vi "main.vi"() -> ()   [LabVIEW 2019]
doc: "This example performs writes and reads on a serial port, as directed by the user. You can press the Write and Read buttons, and change the Read Count, while the example is running.\n\nThe parameters set for the serial port must match the parameters of the connected instrument or device. In this example, the Read Count parameter specifies the number of bytes that the serial port reads. If there were more bytes at the port than the specified number, those bytes would not be read. If there were less bytes at the port than the specified number, you would receive a timeout error.\n\nThis example expands upon the flow control options for XON and XOFF, allowing the user to choose those control characters. Also, the user can enable or disable a termination character. Some devices require a termination character in order to identify the end of command strings. Some devices send a termination character to signify the end of data to be read. This example shows how you can end the Read operation once a termination character is detected in the buffer and/or append a termination character at the end of the Write data."
uses:
  type_cmd.ctl
  type_rxmsg.ctl
panel:
  out "Array":T1[](array[typedef])
  out "stopped":bool=TRUE
  in  "mac2connect":u8[](array[numeric])=[135, 0, 48, 218, 24, 0] format="0x%x"
  in  "cmd":bool
  out "raw cmd":string
  in  "payload":u8[](array[numeric])=[65, 66, 67, 68] format="0x%x"
  in  "command":T2=enum."connect"
  in  "Stop":bool
  in  "VISA resource name":refnum<visa-resource-name>="COM1"
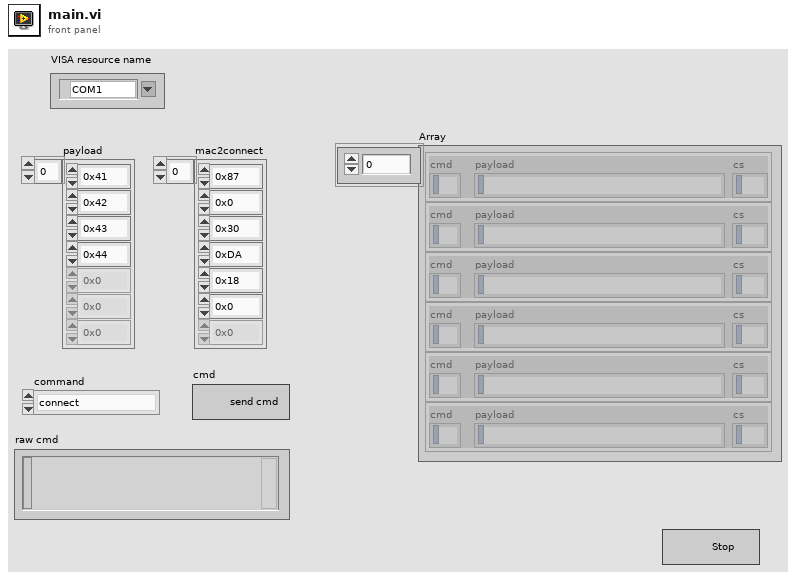
[diagram p1: front panel]
types:
  T1 = typedef "type_rxmsg.ctl" = cluster{"cmd":string, "payload":string, "cs":string}
  T2 = typedef "type_cmd.ctl" = enum16{"setting_factoryreset", "setting_justworks", "scan_getdevices", "scan_stop", "scan_start", "send", "disconnect", "connect"}
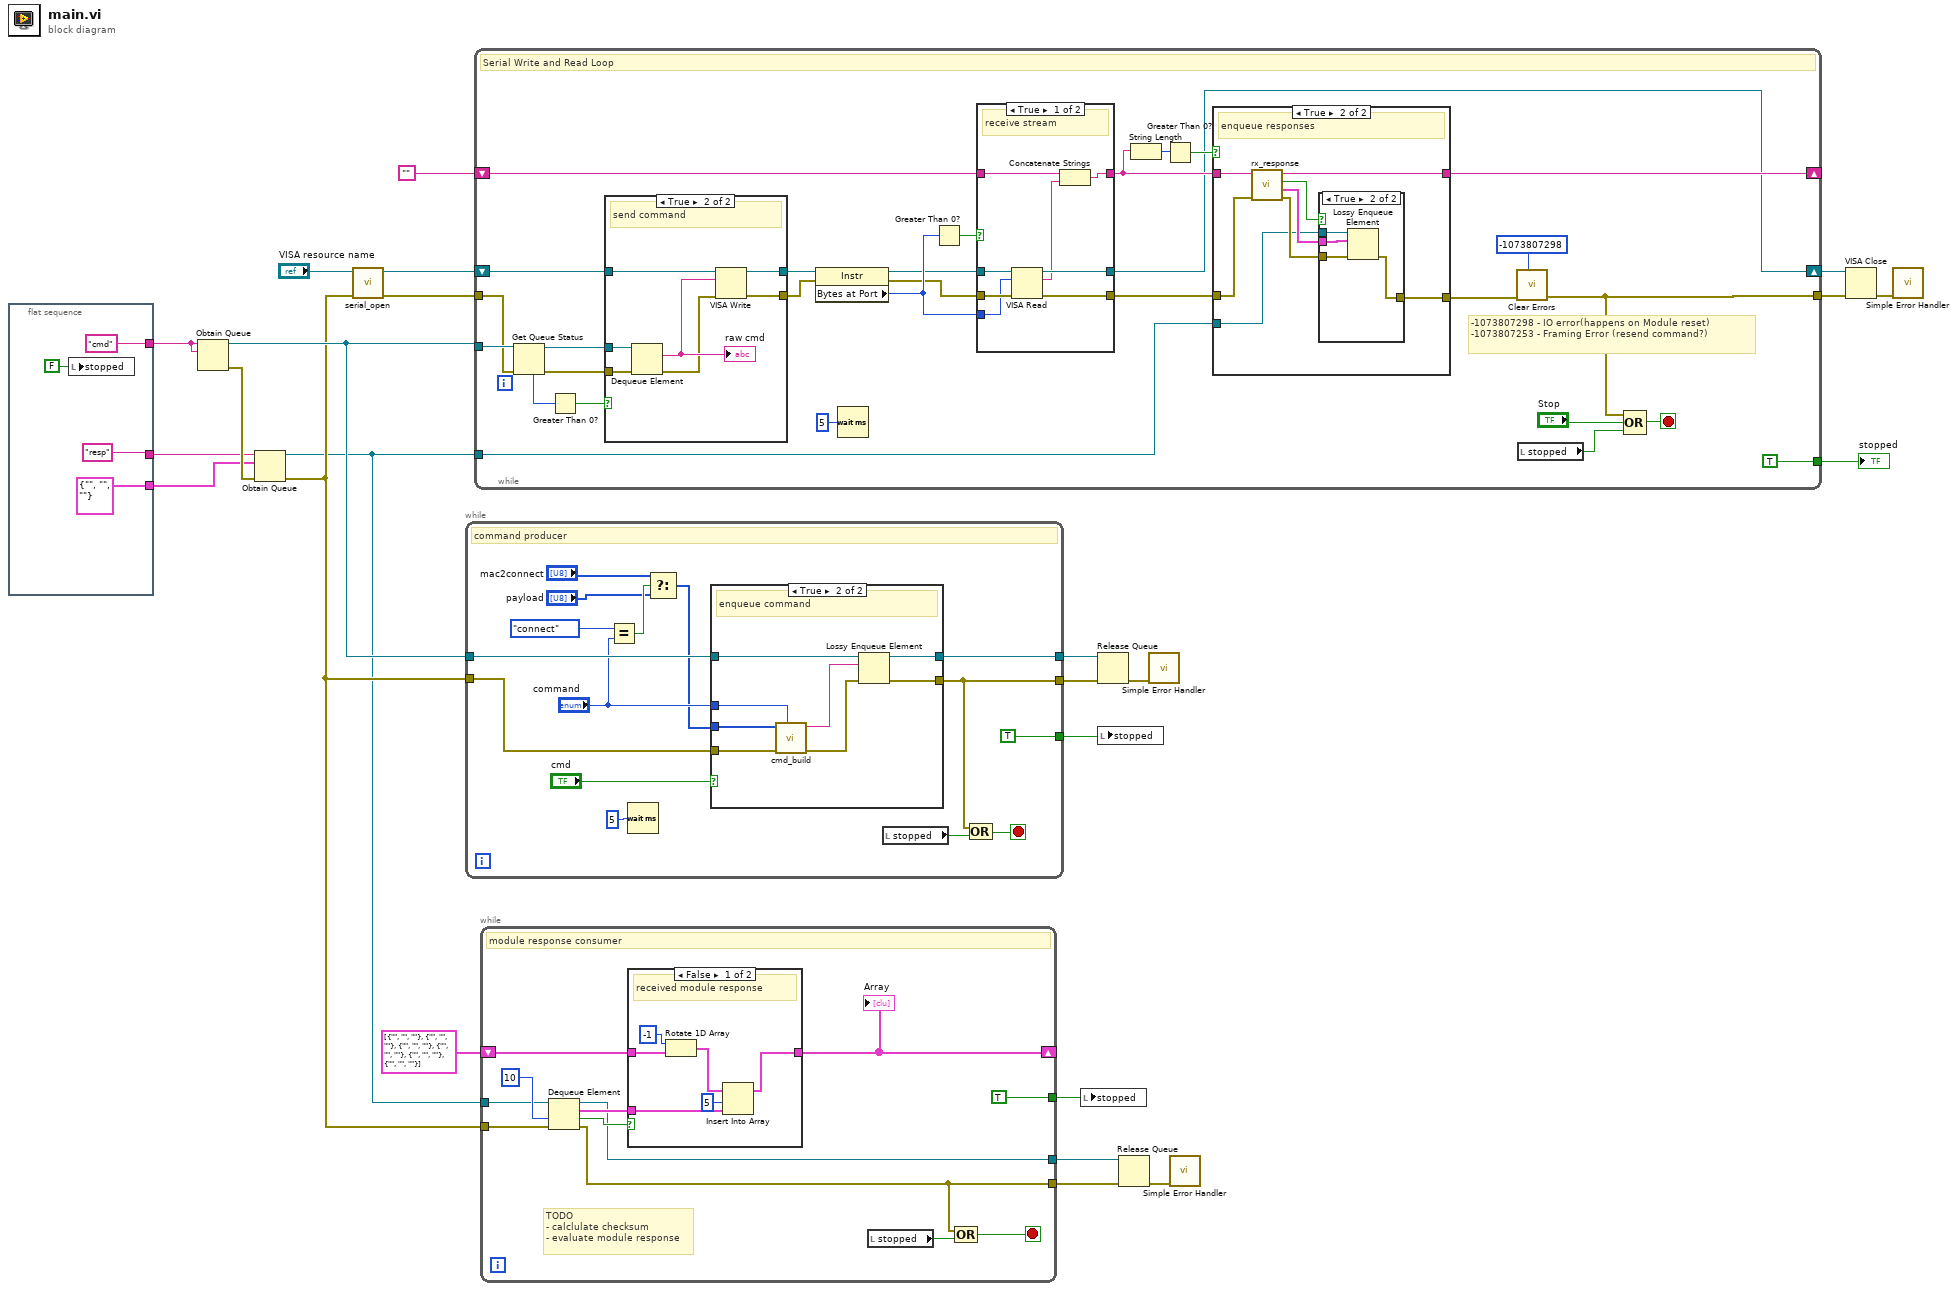
[diagram p0: block diagram]
diagram:
  n1 = flat-sequence {
    tunnel: ["cmd" ("name (unnamed)")] -> w11
    tunnel: ["resp" ("name (unnamed)")] -> w9
    tunnel: [T1 {"cmd"="", "payload"="", "cs"=""} ("rx msg")] -> w8
    frame #0 {
      n2 = local write "stopped"(FALSE ("stopped")) -> ()
    }
  }
  n3 = Obtain Queue(name (unnamed)=w11, element data type=w11) -> (queue out=w15:refnum<queue>, error out=w10:errorcluster)  [unwired: 3 in, 1 out]
  n4 = Obtain Queue(name (unnamed)=w9, element data type=w8, error in (no error)=w10) -> (queue out=w6:refnum<queue>, error out=w7:errorcluster)  [unwired: 2 in, 1 out]
  n5 = call "serial_open.vi"("error in"=w7, "VISA Refnum in"="VISA resource name") -> ("error out"=w20:errorcluster, "VISA Refnum out"=w19:refnum<visa-resource-name>)  [unwired: 8 in]
  n6 = while {
    tunnel: w15 -> [w43]
    tunnel: [w42] -> w18
    tunnel: [w31] -> w17
    tunnel: w7 -> [w41]
    tunnel: [TRUE] -> w12
    stop <- w32 stop-if-true
    # "command producer"
    n7 = Equal?(x=type_cmd."connect" ("command"), y="command") -> (x = y?=w36:bool)
    n8 = Wait (ms)(milliseconds to wait=u32 5) -> ()  [unwired: 1 out]
    n9 = Select(t="mac2connect", s=w36, f="payload") -> (s? t:f=w33:u8[])
    n10 = case shown="True" "cmd" {
      tunnel: w43 -> [w45 w52]
      tunnel: [w45 w53] -> w42
      tunnel: "command" -> [_ w50]
      tunnel: [w44 w48] -> w31
      tunnel: w41 -> [w44 w47]
      tunnel: w33 -> [_ w46]
      frame False {
      }
      frame True {
        # "enqueue command"
        n11 = call "cmd_build.vi"("command"=w50, "error  in"=w47, "payload"=w46) -> ("out"=w49:errorcluster, "cmd"=w51:string)  [unwired: 7 in]
        n12 = Lossy Enqueue Element(queue=w52, element=w51, error in (no error)=w49) -> (queue out=w53:refnum<queue>, error out=w48:errorcluster)  [unwired: 2 out]
      }
    }
    n13 = local read "stopped"() -> (w30:bool)
    n14 = Compound Arithmetic op=OR(w31, w30) -> (w32:bool)
  }
  n15 = while {
    shift-right: [w54] -> w21
    shift-left: w19 -> [w82]
    tunnel: w20 -> [w73]
    tunnel: [w66] -> w22
    tunnel: w15 -> [w77]
    tunnel: [TRUE] -> w14
    shift-right: [w55] -> _
    shift-left: "" -> [w62]
    tunnel: w6 -> [w57]
    stop <- w63 stop-if-true
    # "-1073807298 - IO error(happens on Module reset)\n-1073807253 - Framing Error (resend command?)"
    # "Serial Write and Read Loop"
    n16 = Get Queue Status(queue=w77, error in (no error)=w73) -> (queue out=w74:refnum<queue>, error out=w72:errorcluster, # elements in queue=w76:i32)  [unwired: 1 in, 5 out]
    n17 = Greater Than 0?(x=w76) -> (x > 0?=w75:bool)
    n18 = case shown="True" w75 {
      tunnel: w82 -> [w99 w106]
      tunnel: [w99 w105] -> w69
      tunnel: [w98 w104] -> w71
      tunnel: w74 -> [_ w103]
      tunnel: w72 -> [w98 w101]
      frame False {
      }
      frame True {
        # "send command"
        n19 = Dequeue Element(queue=w103, error in (no error)=w101) -> (element=w102:string, error out=w100:errorcluster)  [unwired: 1 in, 2 out]
        "raw cmd" <- w102
        n20 = VISA Write(VISA resource name=w106, write buffer=w102, error in (no error)=w100) -> (VISA resource name out=w105:refnum<visa-resource-name>, error out=w104:errorcluster)  [unwired: 1 out]
      }
    }
    n21 = property class="Instr"(reference=w69, error in=w71) -> (reference out=w68:refnum<visa-resource-name>, error out=w70:errorcluster, "Bytes at Port"=w79:u32)
    n22 = Wait (ms)(milliseconds to wait=u32 5) -> ()  [unwired: 1 out]
    n23 = Greater Than 0?(x=w79) -> (x > 0?=w80:bool)
    n24 = case shown="True" w80 {
      tunnel: [w112 w117] -> w54
      tunnel: w68 -> [w114 w117]
      tunnel: w70 -> [w113 w115]
      tunnel: w79 -> [w111 _]
      tunnel: w62 -> [w110 w116]
      tunnel: [w108 w116] -> w60
      tunnel: [w107 w115] -> w61
      frame True {
        # "receive stream"
        n25 = VISA Read(VISA resource name=w114, byte count=w111, error in (no error)=w113) -> (VISA resource name out=w112:refnum<visa-resource-name>, read buffer=w109:string, error out=w107:errorcluster)  [unwired: 1 out]
        n26 = Concatenate Strings(w110, w109) -> (w108:string)
      }
      frame False {
      }
    }
    n27 = String Length(string=w60) -> (length=w59:i32)
    n28 = Greater Than 0?(x=w59) -> (x > 0?=w58:bool)
    n29 = case shown="True" w58 {
      tunnel: [w83 w90] -> w55
      tunnel: w61 -> [w84 w92]
      tunnel: w60 -> [w83 w91]
      tunnel: w57 -> [_ w86]
      tunnel: [w84 w85] -> w56
      frame False {
      }
      frame True {
        # "enqueue responses"
        n30 = call "rx_response.vi"("error in"=w92, "msg in"=w91) -> ("error out"=w87:errorcluster, "rx msg"=w88:T1, "msg complete"=w89:bool, "remain"=w90:string)  [unwired: 6 in]
        n31 = case shown="True" w89 {
          tunnel: w88 -> [_ w97]
          tunnel: w87 -> [w93 w96]
          tunnel: w86 -> [_ w95]
          tunnel: [w93 w94] -> w85
          frame False {
          }
          frame True {
            n32 = Lossy Enqueue Element(queue=w95, element=w97, error in (no error)=w96) -> (error out=w94:errorcluster)  [unwired: 3 out]
          }
        }
      }
    }
    n33 = call <vilib>:"Clear Errors.vi"("error in (no error)"=w56, "specific error code to clear (0: all)"=-1073807298) -> ("error out"=w66:errorcluster)  [unwired: 4 in, 1 out]
    n34 = local read "stopped"() -> (w64:bool)
    n35 = Compound Arithmetic op=OR(w66, "Stop", w64) -> (w63:bool)
  }
  "stopped" <- w14
  n36 = while {
    tunnel: w7 -> [w127]
    tunnel: w6 -> [w126]
    shift-right: [w123] -> _
    shift-left: T1[] [{"cmd"="", "payload"="", "cs"=""}, {"cmd"="", "payload"="", "cs"=""}, {"cmd"="", "payload"="", "cs"=""}, {"cmd"="", "payload"="", "cs"=""}, {"cmd"="", "payload"="", "cs"=""}, {"cmd"="", "payload"="", "cs"=""}] -> [w124]
    tunnel: [w121] -> w3
    tunnel: [w120] -> w2
    tunnel: [TRUE] -> w1
    stop <- w119 stop-if-true
    # "TODO \n- calclulate checksum\n- evaluate module response"
    # "module response consumer"
    n37 = Dequeue Element(queue=w126, timeout in ms (-1)=10, error in (no error)=w127) -> (queue out=w121:refnum<queue>, element=w122:T1, timed out?=w125:bool, error out=w120:errorcluster)
    n38 = case shown="False" w125 {
      tunnel: w124 -> [w135 w136]
      tunnel: [w131 w136] -> w123
      tunnel: w122 -> [w130 _]
      frame False {
        # "received module response"
        n39 = Rotate 1D Array(1:w135, 2:-1 ("n")) -> (0:w132:T1[])
        n40 = Insert Into Array(array=w132, index=5, new element=w130) -> (w131:T1[])
      }
      frame True {
      }
    }
    "Array" <- w123
    n41 = local read "stopped"() -> (w128:bool)
    n42 = Compound Arithmetic op=OR(w120, w128) -> (w119:bool)
  }
  n43 = local write "stopped"(w1) -> ()
  n44 = Release Queue(queue=w18, error in (no error)=w17) -> (error out=w16:errorcluster)  [unwired: 1 in, 2 out]
  n45 = local write "stopped"(w12) -> ()
  n46 = Release Queue(queue=w3, error in (no error)=w2) -> (error out=w4:errorcluster)  [unwired: 1 in, 2 out]
  n47 = call <vilib>:"Simple Error Handler.vi"("error in (no error)"=w16) -> ()  [unwired: 1 in, 8 out]
  n48 = call <vilib>:"Simple Error Handler.vi"("error in (no error)"=w4) -> ()  [unwired: 1 in, 8 out]
  n49 = VISA Close(VISA resource name=w21, error in (no error)=w22) -> (error out=w23:errorcluster)
  n50 = call <vilib>:"Simple Error Handler.vi"("error in (no error)"=w23) -> ()  [unwired: 1 in, 8 out]
